vi "PalmSense Read.vi"(8 "error in (no error)":errorcluster, 9 "Message Data":variant, 11 "Hardware Resources in":T1) -> (0 "error out":errorcluster, 1 "Message Data Out":variant, 3 "Hardware Resources out":T1)   [LabVIEW 2020, in "PalmSens.lvlib"]
doc: "Perform the acquisition. Replace the contents of this diagram with calls to acquisition hardware."
uses:
  PalmSens.lvlib
  PalmSense Hardware Configuration.ctl
  <instrlib>/PalmSens SDK for LabVIEW 5.10/PalmSens/PalmSens.lvclass
  support/Message Queue/Message Cluster.ctl
  support/Message Queue/Message Queue.lvlib
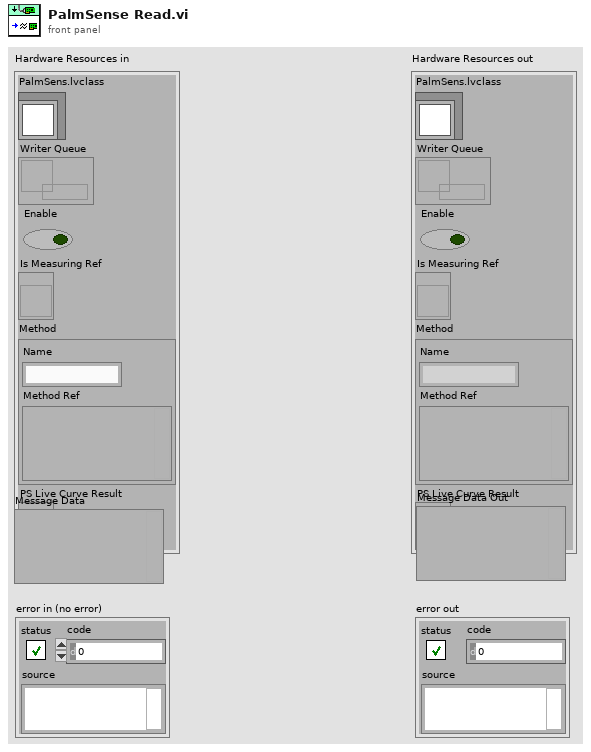
[diagram p1: front panel]
types:
  T1 = typedef "PalmSens.lvlib/PalmSense Hardware Configuration.ctl" = cluster{"PalmSens.lvclass":refnum<class "PalmSens.lvclass">, "Writer Queue":refnum<queue>, "Enable":bool, "Is Measuring Ref":refnum<vi>, "Method":cluster{"Name":string, "Method Ref":variant}, "PS Live Curve Result":refnum<vi>}
  T2 = typedef "Message Queue.lvlib/Message Cluster.ctl" = cluster{"Message":string, "Message Data":variant}
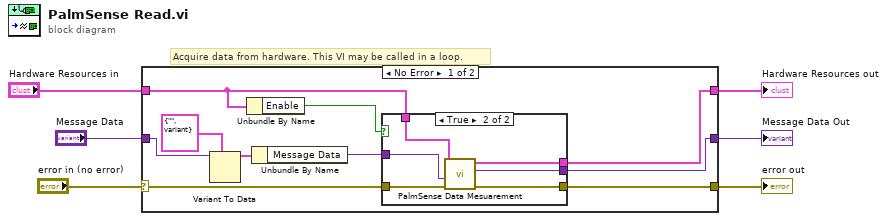
[diagram p0: block diagram]
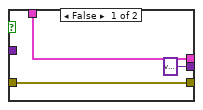
[diagram p2: hidden frame]
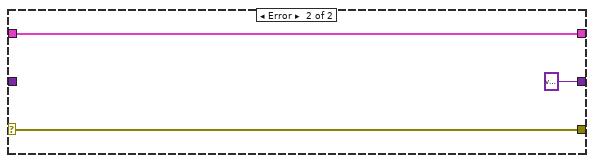
[diagram p3: hidden frame]
diagram:
  # "Acquire data from hardware. This VI may be called in a loop."
  n1 = case shown="No Error" "error in (no error)" {
    selector: "error in (no error)" -> [w10 w27]
    tunnel: [w15 w27] -> w5
    tunnel: "Hardware Resources in" -> [w8 w28]
    tunnel: [w16 w28] -> w3
    tunnel: [w14 variant ("Message Data Out")] -> w2
    tunnel: "Message Data" -> [w12 _]
    frame No Error {
      n2 = Variant To Data(type=T2 {"Message"="", "Message Data"=variant} ("element"), Variant=w12) -> (data=w11:T2)  [unwired: 1 in, 1 out]
      n3 = Unbundle By Name(w8) -> ("Enable"=w7:bool)
      n4 = Unbundle By Name(w11) -> ("Message Data"=w9:variant)
      n5 = case shown="True" w7 {
        tunnel: [w19 w25] -> w16
        tunnel: [w18 w24] -> w15
        tunnel: [variant ("Message Data Out") w23] -> w14
        tunnel: w10 -> [w18 w22]
        tunnel: w9 -> [_ w21]
        tunnel: w8 -> [w19 w20]
        frame False {
        }
        frame True {
          n6 = call "PalmSense Data Mesuarement.vi"("error in (no error)"=w22, "Message Data"=w21, "Hardware Resources in"=w20) -> ("error out"=w24:errorcluster, "Message Data Out"=w23:variant, "Hardware Resources out"=w25:T1)  [unwired: 6 in]
        }
      }
    }
    frame Error {
    }
  }
  "Hardware Resources out" <- w3
  "error out" <- w5
  "Message Data Out" <- w2
